vi "TEMP2xxx Control.vi"() -> ()   [LabVIEW 2017]
uses:
  <instrlib>/Samwontech TEMP2xxx/Samwontech TEMP2xxx.lvlib
panel:
  in  "Close port":bool
  in  "Open port":bool
  in  "Exit":bool
  in  "Serial Configuration":T1={"Baud Rate"=9600, "Parity"=0, "Data Bits"=8, "Stop Bits"=10, "Flow Control"=0} {"Flow Control" items=["None", "XON/XOFF", "RTS/CTS", "XON/XOFF & RTS/CTS", "DTR/DSR", "XON/XOFF & DTR/DSR"]; "Stop Bits" items=["1.0"=10, "1.5"=15, "2.0"=20]; "Data Bits" items=["7"=7, "8"=8]; "Parity" items=["None", "Odd", "Even", "Mark", "Space"]; "Baud Rate" items=["300"=300, "600"=600, "1200"=1200, "2400"=2400, "4800"=4800, "9600"=9600, "19200"=19200, "115200"=115200]}
  in  "VISA resource name":refnum<visa-resource-name>
  out "Successfully":bool
  in  "FIX Set Point":dbl format="%1.1f"
  in  "Set Fix Operation Set Point":bool
  out "Successfully":bool
  in  "Run FIX":bool
  in  "Read continuously":bool
  in  "Read Current PV":bool
  out "Data Valid":bool
  out "Current PV":dbl
  out "Responce (original)":string
  out "Successfully":bool
  in  "Data":u32
  in  "Register (write)":u32=1
  in  "Write":bool
  out "Data":u32
  out "Data Valid":bool
  in  "Register (read)":u32=1
  in  "Read":bool
  out "Version-Revision":string
  out "Model Name":string
  in  "AMI":bool
  # "Registers Read/Write:"
  # "FIX Mode Control:"
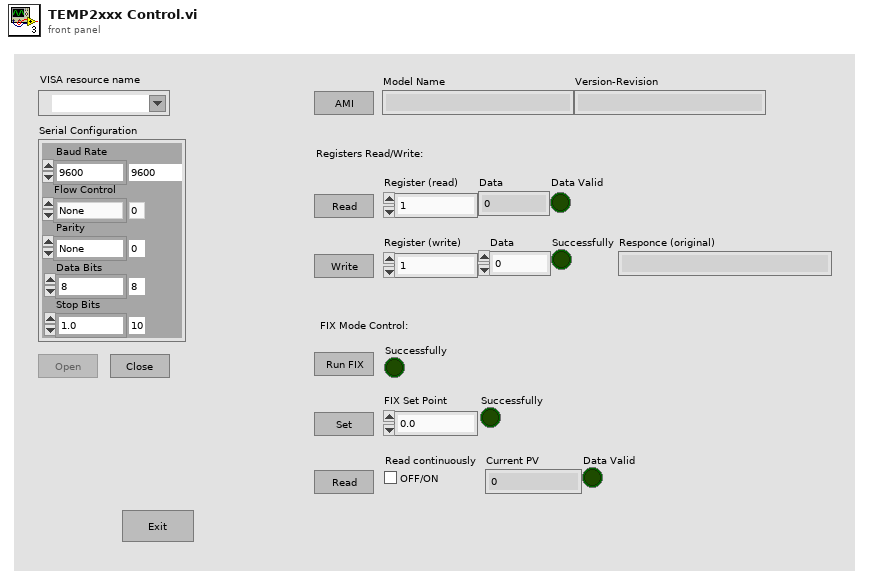
[diagram p1: front panel]
types:
  T1 = cluster{"Baud Rate":u32, "Parity":u16, "Data Bits":u16, "Stop Bits":u16, "Flow Control":u16}
  T2 = enum8{"Enabled", "Disabled", "Disabled and Grayed Out"}
  T3 = enum32{"Invalid", "Standard", "Closed", "Hidden", "Minimized", "Maximized"}
  T4 = enum32{"invalid app kind", "Development System", "Run Time System", "Student Edition", "Embedded LabVIEW", "Evaluation", "Custom"}
  T5 = cluster{"Core":cluster{"Current VI Reference":refnum<vi>, "Close Panel on Exit?":bool}, "Your Boolean data":bool, "Your string data":string, "VISA resource name":refnum<visa-resource-name>, "Is port opened?":bool, "Read: Current PV":bool}
  T6 = cluster{"Current VI Reference":refnum<vi>, "Close Panel on Exit?":bool}
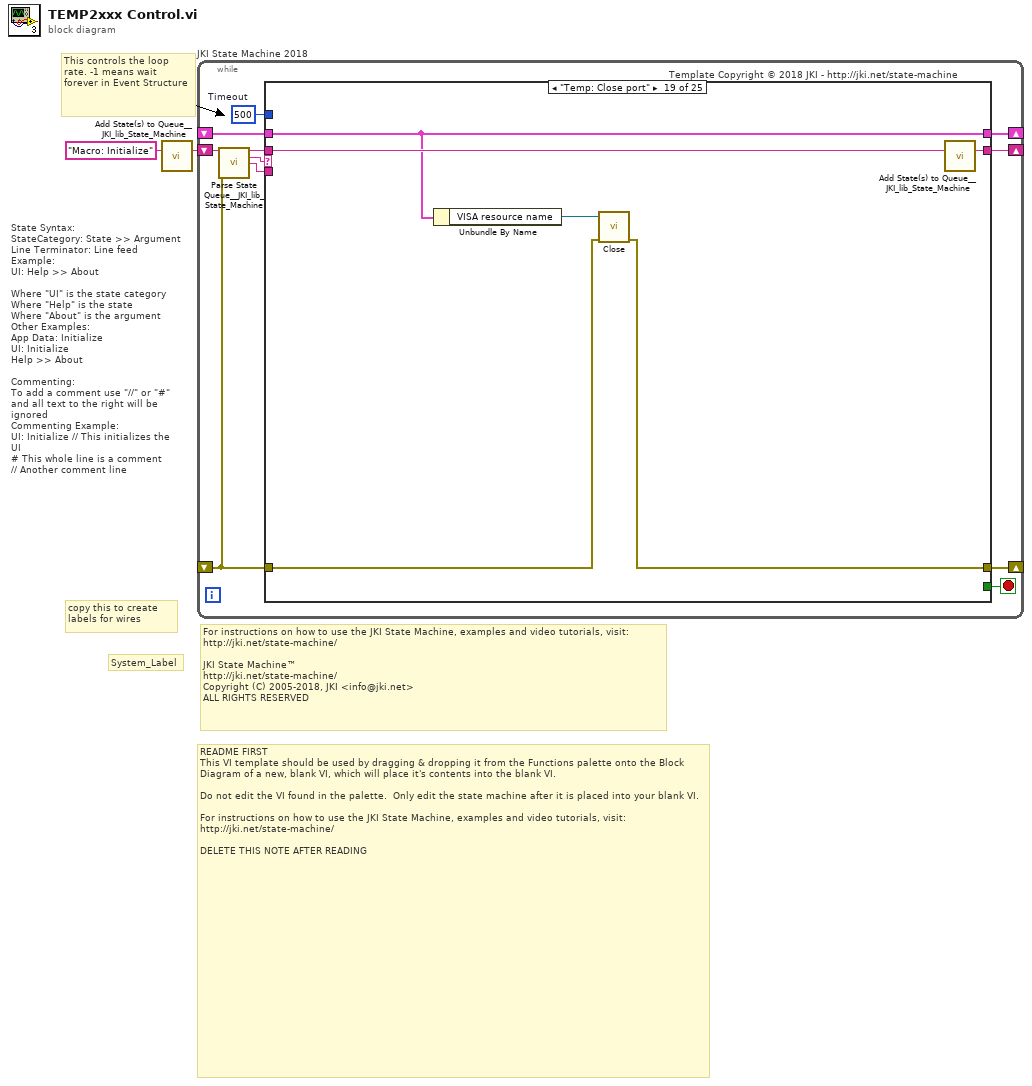
[diagram p0: block diagram]
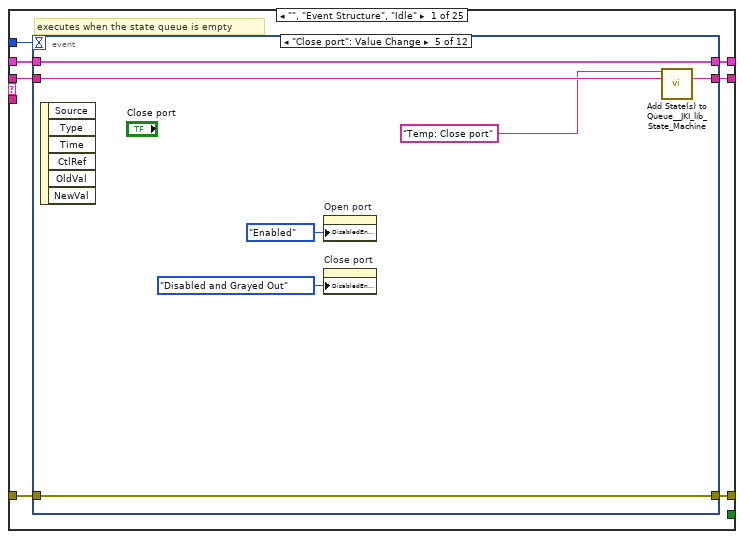
[diagram p2: hidden frame]
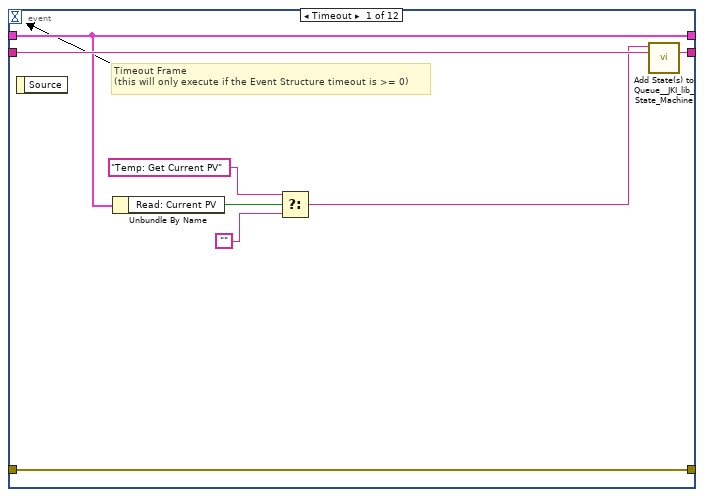
[diagram p3: hidden frame]
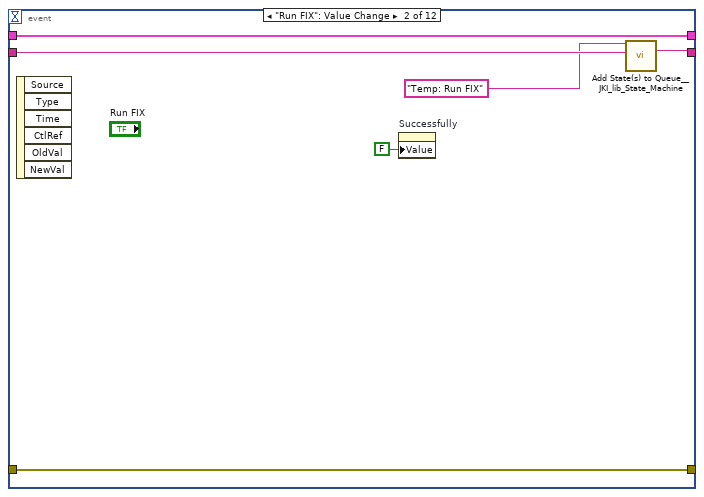
[diagram p4: hidden frame]
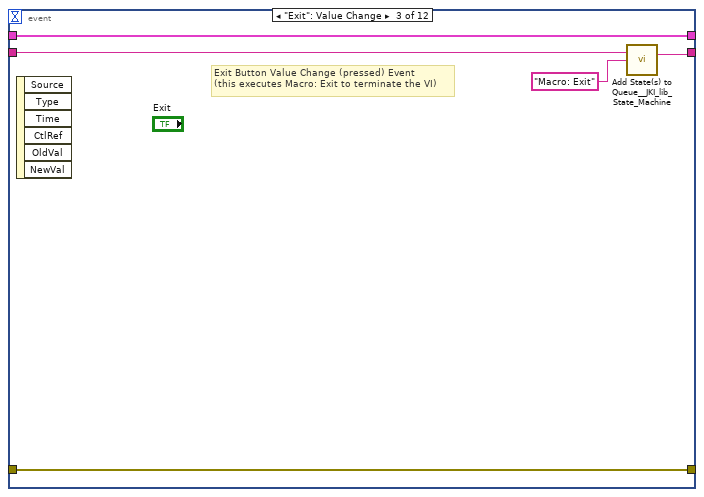
[diagram p5: hidden frame]
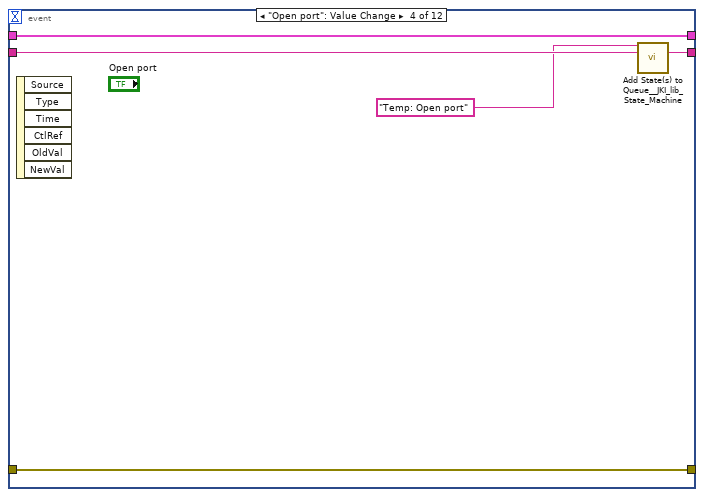
[diagram p6: hidden frame]
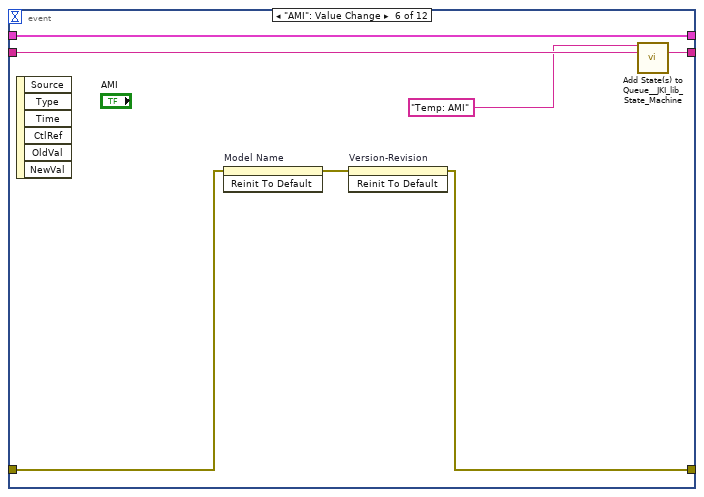
[diagram p7: hidden frame]
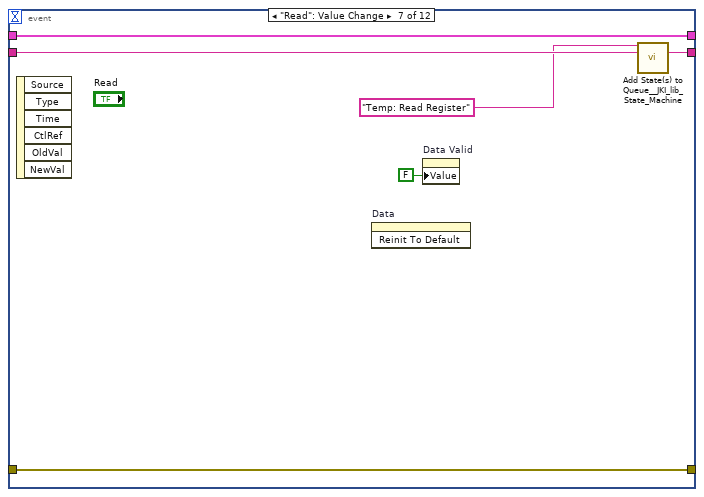
[diagram p8: hidden frame]
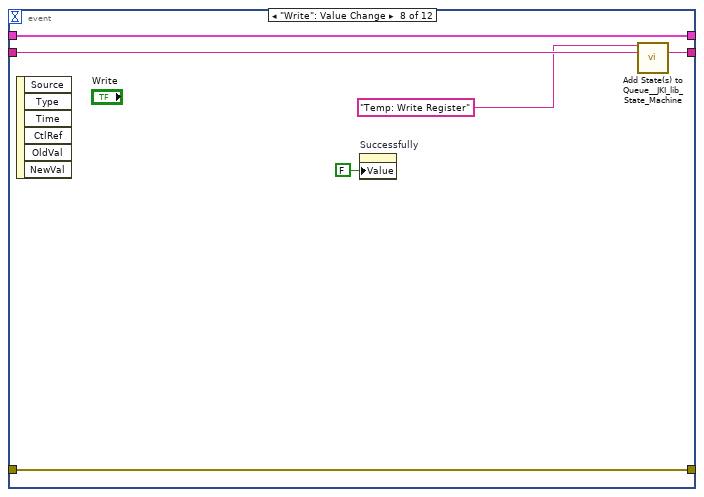
[diagram p9: hidden frame]
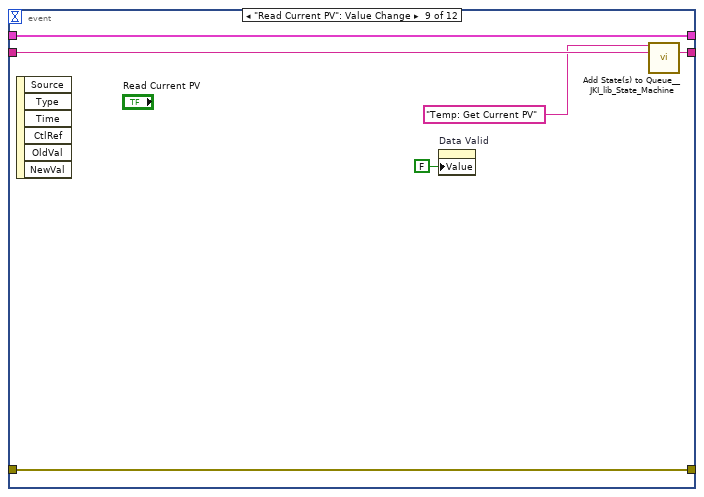
[diagram p10: hidden frame]
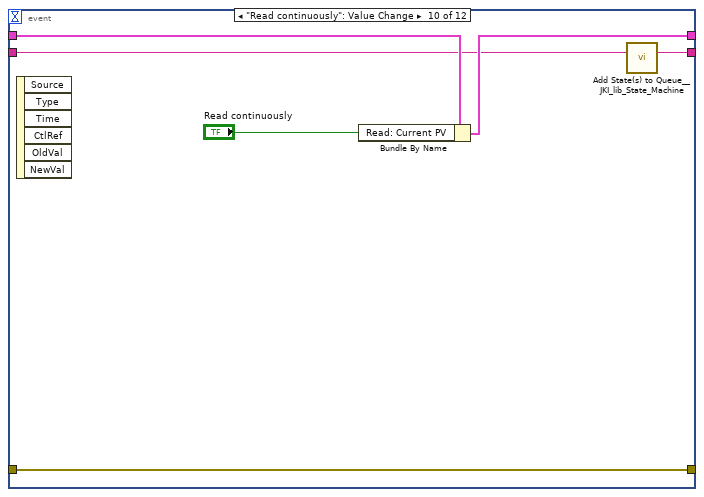
[diagram p11: hidden frame]
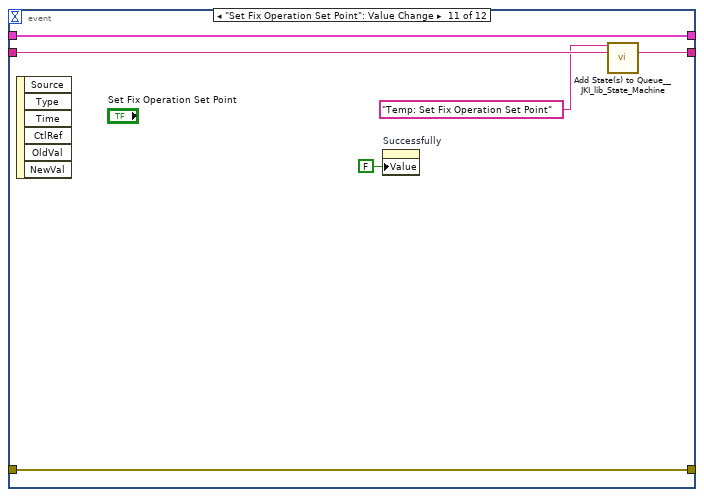
[diagram p12: hidden frame]
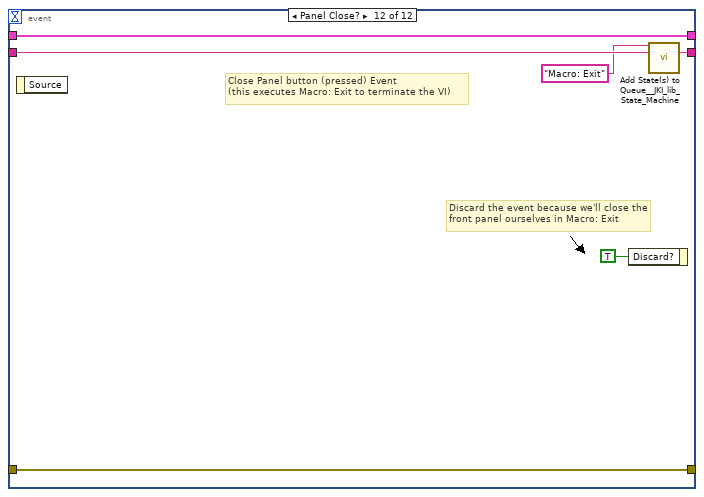
[diagram p13: hidden frame]
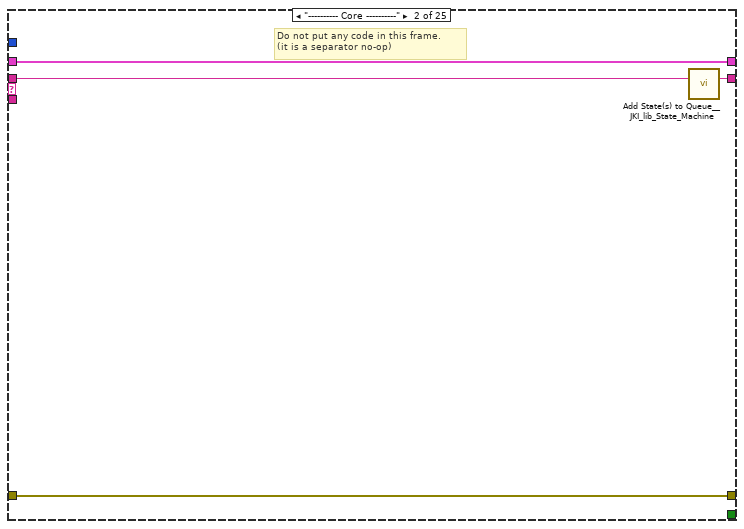
[diagram p14: hidden frame]
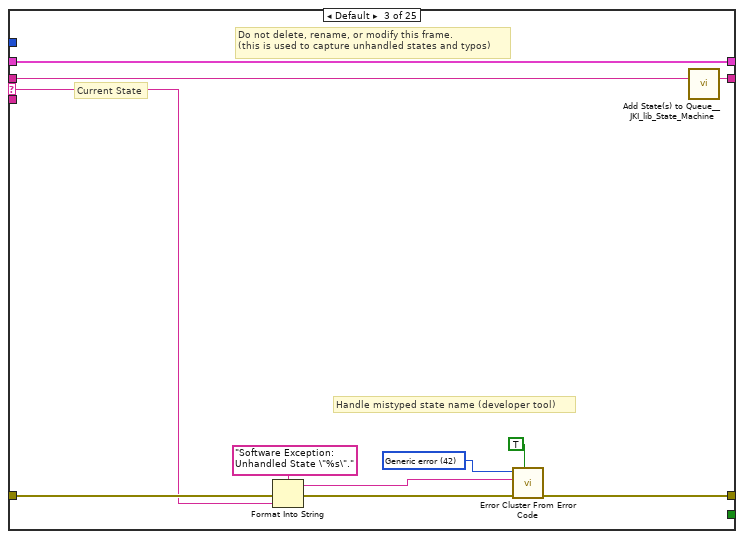
[diagram p15: hidden frame]
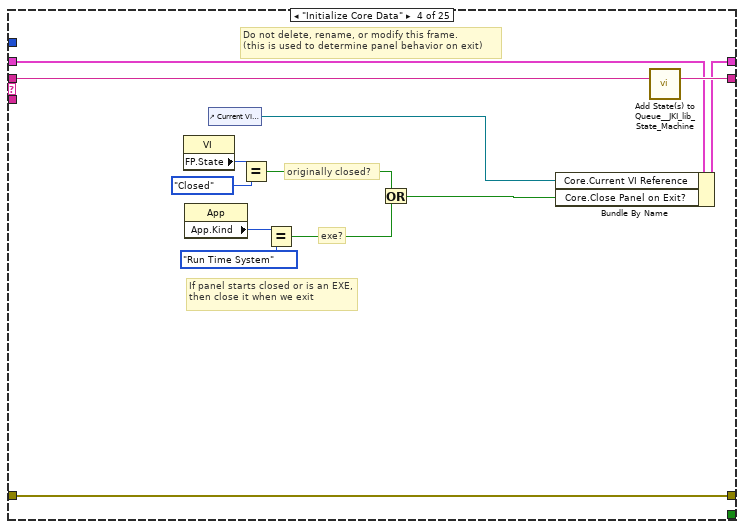
[diagram p16: hidden frame]
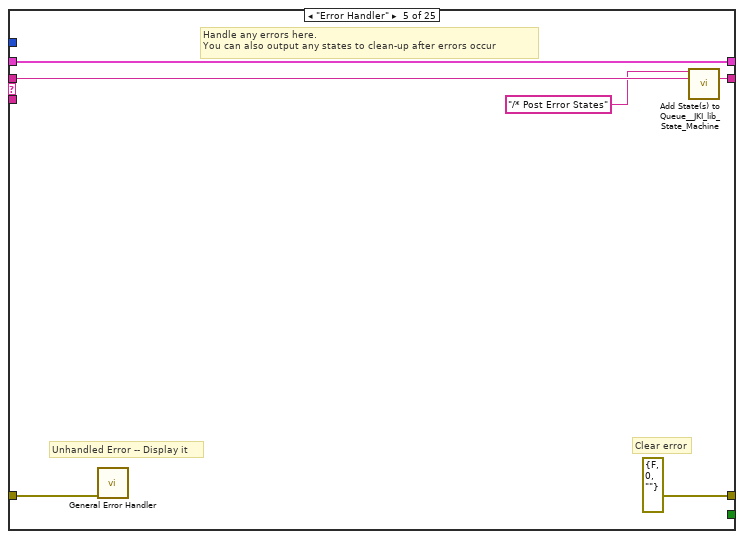
[diagram p17: hidden frame]
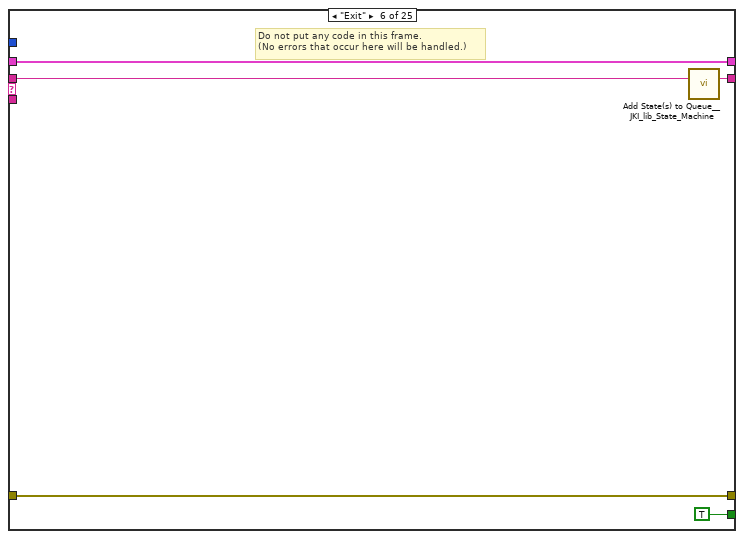
[diagram p18: hidden frame]
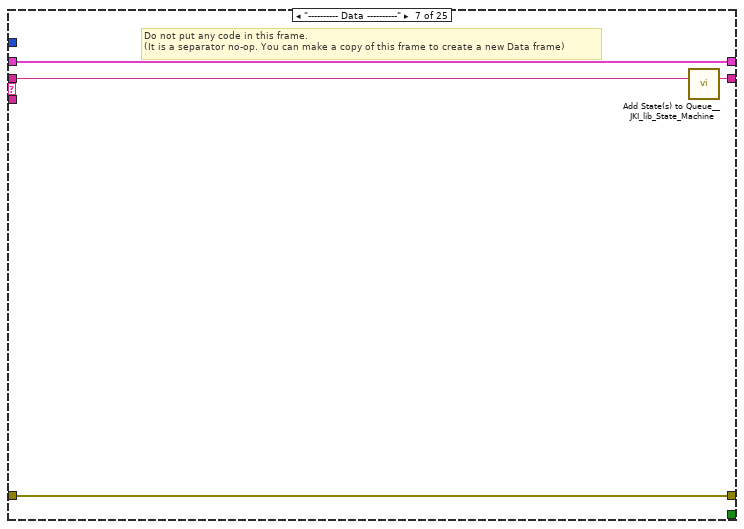
[diagram p19: hidden frame]
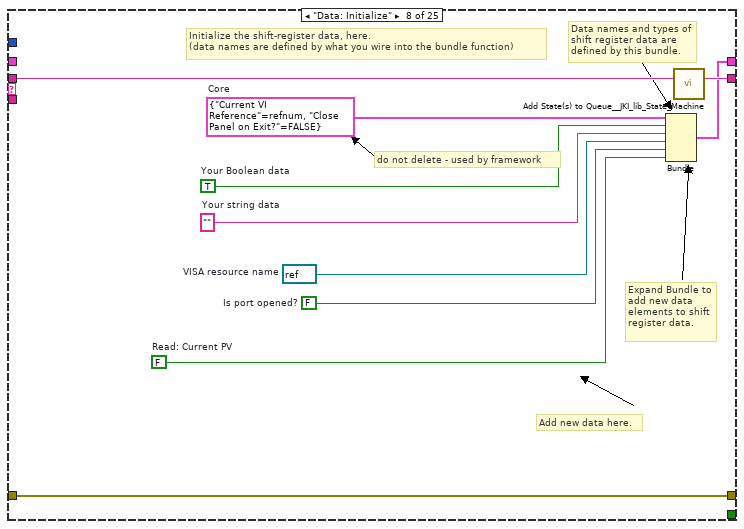
[diagram p20: hidden frame]
diagram:
  # "README FIRST\nThis VI template should be used by dragging & dropping it from the Functions palette onto the Block Diagram of a new, blank VI, which will place it's contents into the blank VI.\n\nDo not edit the VI found in the palette.  Only edit the state machine after it is placed into your blank VI.\n\nFor instructions on how to use the JKI State Machine, examples and video tutorials, visit:\nhttp://jki.net/state-machine/\n\nDELETE THIS NOTE AFTER READING"
  # "For instructions on how to use the JKI State Machine, examples and video tutorials, visit:\nhttp://jki.net/state-machine/\n\nJKI State Machine™\nhttp://jki.net/state-machine/\nCopyright (C) 2005-2018, JKI <info@jki.net>\nALL RIGHTS RESERVED"
  # "State Syntax:\nStateCategory: State >> Argument\nLine Terminator: Line feed\nExample:\nUI: Help >> About\n\nWhere \"UI\" is the state category\nWhere \"Help\" is the state\nWhere \"About\" is the argument\nOther Examples:\nApp Data: Initialize\nUI: Initialize\nHelp >> About\n\nCommenting:\nTo add a comment use \"//\" or \"#\" and all text to the right will be ignored\nCommenting Example:\nUI: Initialize // This initializes the UI\n# This whole line is a comment\n// Another comment line"
  # "copy this to create labels for wires"
  # "This controls the loop rate. -1 means wait forever in Event Structure"
  # "System_Label"
  n1 = call <vilib>:"Add State(s) to Queue__JKI_lib_State_Machine.vi"("State(s) in (\"\")"="Macro: Initialize") -> ("States Out"=w2:string)  [unwired: 14 in]
  n2 = while "JKI State Machine 2018" {
    shift-right: [w6] -> _
    shift-left: _ -> [w5]
    shift-right: [w9] -> _
    shift-left: _ -> [w3]
    shift-right: [w8] -> _
    shift-left: w2 -> [w10]
    stop <- w7 stop-if-true
    w4 = 500  # Timeout
    # "Template Copyright © 2018 JKI - http://jki.net/state-machine"
    n3 = call <vilib>:"Parse State Queue__JKI_lib_State_Machine.vi"("State Queue"=w10, "Error In (no error)"=w3) -> ("Remaining States"=w12:string, "Current State"=w13:string, "Arguments"=w11:string)  [unwired: 11 in]
    n4 = case shown="\"Temp: Close port\"" w13 {
      selector: w13 -> [_ _ w99 _ _ _ _ _ _ _ _ _ _ _ _ _ _ _ _ _ _ _ _ _ _]
      tunnel: w12 -> [w20 w98 w103 w122 w128 w133 w137 w147 w153 w157 w163 w169 w180 w249 w254 w266 w274 w286 w294 w302 w311 w321 w329 w336 w344]
      tunnel: w11 -> [_ _ _ _ _ _ _ _ _ _ _ w164 w174 _ _ _ _ _ _ _ _ _ _ _ _]
      tunnel: w5 -> [w18 w95 w101 w115 w125 w131 w134 _ w148 w154 w161 w167 w176 w246 w251 w263 w271 w281 w292 w300 w309 w319 w327 w334 w342]
      tunnel: [w17 w96 w105 w119 errorcluster {"status"=FALSE, "code"=0, "source"=""} ("error out") w130 w135 w144 w149 w155 w160 w165 w177 w247 w252 w264 w272 w277 w289 w297 w305 w314 w324 w331 w338] -> w9
      tunnel: w3 -> [w16 w96 w104 w119 w124 w130 w135 w144 w150 w155 w160 w166 w178 w247 w252 w264 w272 w279 w290 w298 w306 w315 w325 w332 w339]
      tunnel: [w19 w97 w102 w121 w127 w132 w136 w146 w152 w156 w162 w168 w179 w248 w253 w265 w273 w285 w293 w301 w310 w320 w328 w335 w343] -> w8
      tunnel: [_ _ _ _ _ TRUE _ _ _ _ _ _ _ _ _ _ _ _ _ _ _ _ _ _ _] -> w7
      tunnel: [w15 w95 w101 w120 w125 w131 w134 w145 w148 w154 w161 w167 w176 w246 w251 w263 w271 w280 w292 w300 w309 w319 w327 w334 w342] -> w6
      tunnel: w4 -> [w14 _ _ _ _ _ _ _ _ _ _ _ _ _ _ _ _ _ _ _ _ _ _ _ _]
      frame "", "Event Structure", "Idle" {
        # "executes when the state queue is empty"
        n5 = event shown="[4] \"Close port\": Value Change" {
          selector: _ -> [_ _ _ _ _ _ _ _ _ _ _ _]
          dyn-events: _ -> [_ _ _ _ _ _ _ _ _ _ _ _]
          timeout: w14 -> [_ _ _ _ _ _ _ _ _ _ _ _]
          tunnel: w20 -> [w28 w31 w36 w41 w48 w56 w61 w67 w75 w78 w85 w94]
          tunnel: [w27 w32 w37 w42 w49 w57 w62 w68 w74 w79 w86 w93] -> w19
          tunnel: w18 -> [w25 w33 w38 w43 w50 w58 w63 w69 w76 w81 w87 w91]
          tunnel: [w26 w34 w39 w44 w51 w52 w64 w70 w73 w82 w88 w92] -> w17
          tunnel: w16 -> [w26 w34 w39 w44 w51 w54 w64 w70 w73 w82 w88 w92]
          tunnel: [w25 w33 w38 w43 w50 w58 w63 w69 w76 w80 w87 w91] -> w15
          event Timeout {
            # "Timeout Frame\n(this will only execute if the Event Structure timeout is >= 0)"
            n6 = event-data() -> ()  [unwired: 1 in, 1 out]
            n7 = Unbundle By Name(w25) -> ("Read: Current PV"=w24:bool)
            n8 = Select(t="Temp: Get Current PV", s=w24, f="") -> (s? t:f=w21:string)
            n9 = call <vilib>:"Add State(s) to Queue__JKI_lib_State_Machine.vi"("State(s) in Front (\"\")"=w21, "State(s) in (\"\")"=w28) -> ("States Out"=w27:string)  [unwired: 13 in]
          }
          event "Run FIX": Value Change {
            n10 = event-data() -> ()  [unwired: 1 in, 6 out]
            n11 = property on="Successfully" class="Bool (strict)"("Value"=FALSE ("Successfully")) -> ()  [unwired: 2 in, 2 out]
            n12 = call <vilib>:"Add State(s) to Queue__JKI_lib_State_Machine.vi"("State(s) in Front (\"\")"="Temp: Run FIX", "State(s) in (\"\")"=w31) -> ("States Out"=w32:string)  [unwired: 13 in]
          }
          event "Exit": Value Change {
            # "Exit Button Value Change (pressed) Event\n(this executes Macro: Exit to terminate the VI)"
            n13 = event-data() -> ()  [unwired: 1 in, 6 out]
            n14 = call <vilib>:"Add State(s) to Queue__JKI_lib_State_Machine.vi"("State(s) in (\"\")"=w36, "State(s) at Back (\"\")"="Macro: Exit" ("State(s) at Back (\"\")")) -> ("States Out"=w37:string)  [unwired: 13 in]
          }
          event "Open port": Value Change {
            n15 = event-data() -> ()  [unwired: 1 in, 6 out]
            n16 = call <vilib>:"Add State(s) to Queue__JKI_lib_State_Machine.vi"("State(s) in Front (\"\")"="Temp: Open port" ("State(s) in Front (\"\")"), "State(s) in (\"\")"=w41) -> ("States Out"=w42:string)  [unwired: 13 in]
          }
          event "Close port": Value Change {
            n17 = event-data() -> ()  [unwired: 1 in, 6 out]
            n18 = property on="Open port" class="Bool"("DisabledEnum"=T2."Enabled" ("Disabled")) -> ()  [unwired: 2 in, 2 out]
            n19 = property on="Close port" class="Bool"("DisabledEnum"=T2."Disabled and Grayed Out" ("Disabled")) -> ()  [unwired: 2 in, 2 out]
            n20 = call <vilib>:"Add State(s) to Queue__JKI_lib_State_Machine.vi"("State(s) in Front (\"\")"="Temp: Close port" ("State(s) in Front (\"\")"), "State(s) in (\"\")"=w48) -> ("States Out"=w49:string)  [unwired: 13 in]
          }
          event "AMI": Value Change {
            n21 = event-data() -> ()  [unwired: 1 in, 6 out]
            n22 = invoke on="Model Name" class="Str" method="Reinit To Default"(error in=w54) -> (error out=w53:errorcluster)  [unwired: 2 in, 2 out]
            n23 = invoke on="Version-Revision" class="Str" method="Reinit To Default"(error in=w53) -> (error out=w52:errorcluster)  [unwired: 2 in, 2 out]
            n24 = call <vilib>:"Add State(s) to Queue__JKI_lib_State_Machine.vi"("State(s) in Front (\"\")"="Temp: AMI" ("State(s) in Front (\"\")"), "State(s) in (\"\")"=w56) -> ("States Out"=w57:string)  [unwired: 13 in]
          }
          event "Read": Value Change {
            n25 = event-data() -> ()  [unwired: 1 in, 6 out]
            n26 = invoke on="Data" class="DigNum (strict)" method="Reinit To Default"() -> ()  [unwired: 3 in, 3 out]
            n27 = property on="Data Valid" class="Bool (strict)"("Value"=FALSE ("Data Valid")) -> ()  [unwired: 2 in, 2 out]
            n28 = call <vilib>:"Add State(s) to Queue__JKI_lib_State_Machine.vi"("State(s) in Front (\"\")"="Temp: Read Register" ("State(s) in Front (\"\")"), "State(s) in (\"\")"=w61) -> ("States Out"=w62:string)  [unwired: 13 in]
          }
          event "Write": Value Change {
            n29 = event-data() -> ()  [unwired: 1 in, 6 out]
            n30 = property on="Successfully" class="Bool (strict)"("Value"=FALSE ("Successfully")) -> ()  [unwired: 2 in, 2 out]
            n31 = call <vilib>:"Add State(s) to Queue__JKI_lib_State_Machine.vi"("State(s) in Front (\"\")"="Temp: Write Register" ("State(s) in Front (\"\")"), "State(s) in (\"\")"=w67) -> ("States Out"=w68:string)  [unwired: 13 in]
          }
          event "Read Current PV": Value Change {
            n32 = event-data() -> ()  [unwired: 1 in, 6 out]
            n33 = property on="Data Valid" class="Bool (strict)"("Value"=FALSE ("Data Valid")) -> ()  [unwired: 2 in, 2 out]
            n34 = call <vilib>:"Add State(s) to Queue__JKI_lib_State_Machine.vi"("State(s) in Front (\"\")"="Temp: Get Current PV" ("State(s) in Front (\"\")"), "State(s) in (\"\")"=w75) -> ("States Out"=w74:string)  [unwired: 13 in]
          }
          event "Read continuously": Value Change {
            n35 = event-data() -> ()  [unwired: 1 in, 6 out]
            n36 = Bundle By Name(cluster=w81, "Read: Current PV"="Read continuously") -> (w80:T5)
            n37 = call <vilib>:"Add State(s) to Queue__JKI_lib_State_Machine.vi"("State(s) in (\"\")"=w78) -> ("States Out"=w79:string)  [unwired: 14 in]
          }
          event "Set Fix Operation Set Point": Value Change {
            n38 = event-data() -> ()  [unwired: 1 in, 6 out]
            n39 = property on="Successfully" class="Bool (strict)"("Value"=FALSE ("Successfully")) -> ()  [unwired: 2 in, 2 out]
            n40 = call <vilib>:"Add State(s) to Queue__JKI_lib_State_Machine.vi"("State(s) in Front (\"\")"="Temp: Set Fix Operation Set Point", "State(s) in (\"\")"=w85) -> ("States Out"=w86:string)  [unwired: 13 in]
          }
          event Panel Close? {
            # "Discard the event because we'll close the front panel ourselves in Macro: Exit"
            # "Close Panel button (pressed) Event\n(this executes Macro: Exit to terminate the VI)"
            n41 = event-data() -> ()  [unwired: 1 in, 1 out]
            n42 = event-data("Discard?"=TRUE) -> ()  [unwired: 1 in, 1 out]
            n43 = call <vilib>:"Add State(s) to Queue__JKI_lib_State_Machine.vi"("State(s) in Front (\"\")"="Macro: Exit", "State(s) in (\"\")"=w94) -> ("States Out"=w93:string)  [unwired: 13 in]
          }
        }
      }
      frame "---------- Core ----------" {
        # "Do not put any code in this frame.\n(it is a separator no-op)"
        n44 = call <vilib>:"Add State(s) to Queue__JKI_lib_State_Machine.vi"("State(s) in (\"\")"=w98) -> ("States Out"=w97:string)  [unwired: 14 in]
      }
      frame Default {
        w108 = 42 items=["No error", "Argument error", "Memory is full", "Out of zone", "End of file", "File already open", "Generic file I/O error", "File not found", "File permission error", "Disk is full", "Duplicate path", "Too many files open", "System feature not enabled", "Resource file not found", "Cannot add resource", "Resource not found", "Image not found", "Image memory error", "Pen does not exist", "Config type invalid", "Config token not found", "Config parse error", "Config memory error", "Bad external code format", "Bad external code offset", "External code not present", "Null window", "Destroy window error", "Null menu", "Print aborted", "Bad print record", "Print driver error", "Windows error during printing", "Memory error during printing", "Print dialog error", "Generic print error", "Invalid device refnum", "Device not found", "Device parameter error", "Device unit error", "Cannot open device", "Device call aborted", "Generic error", "Cancelled by user", "Object ID too low", "Object ID too high", "Object not in heap", "Unknown heap", "Unknown object (invalid DefProc)", "Unknown object (DefProc not in table)", "Message out of range", "Invalid (null) method", "Unknown message", "Manager call not supported", "Bad address", "Network operation in progress", "Network operation timed out", "Connection is busy", "Network attribute not supported", "Network error", "Address in use", "System out of memory", "Connection aborted", "Connection refused", "Not connected", "Already connected", "Connection closed", "Initialization error (interapplication manager)", "Bad occurrence", "Wait on unbound occurrence handler", "Occurrence queue overflow", "Datalog type conflict", "Unused", "Unrecognized type (interapplication manager)", "Memory corrupt", "Failed to make temporary DLL", "Old CIN version", "Drag socket not found", "Failed to load drop-object", "Failed to register OLE object", "Failed to release OLE object", "Format specifier type mismatch", "Unknown format specifier", "Too few format specifiers", "Too many format specifiers", "Scan failed", "Newer CIN version", "Error converting to variant", "Runtime menu error", "Password tampered", "Variant attribute not found", "Incompatible variant data type", "Event data is not available", "Event Store is not present", "Occurrence is not found", "Event Queue is not created", "Event info is not available", "Refnum passed is NULL", "Error retrieving Class GUID", "Error retrieving CoClass GUID", "Error retrieving TypeLib GUID.", "Bad built application magic bytes.", "Specific driver is different from the specific driver associated with the Logical Name.", "There is no session opened to the class driver.", "Max Error", "MAX - Error with config objects", "MAX - Error loading configuration", "MAX - Group not supported"]
        # "Current State"
        # "Do not delete, rename, or modify this frame.\n(this is used to capture unhandled states and typos)"
        # "Handle mistyped state name (developer tool)"
        n45 = Format Into String(format string="Software Exception: Unhandled State \"%s\"." ("message"), error in=w104, w99) -> (resulting string=w107:string, error out=w106:errorcluster)  [unwired: 1 in]
        n46 = call <vilib>:"Error Cluster From Error Code.vi"("show call chain? (False)"=TRUE, "error in (no error)"=w106, "error message (\"\")"=w107, "error code (0)"=w108) -> ("error out"=w105:errorcluster)  [unwired: 5 in]
        n47 = call <vilib>:"Add State(s) to Queue__JKI_lib_State_Machine.vi"("State(s) in (\"\")"=w103) -> ("States Out"=w102:string)  [unwired: 14 in]
      }
      frame "Initialize Core Data" {
        # "Do not delete, rename, or modify this frame.\n(this is used to determine panel behavior on exit)"
        # "originally closed?"
        # "exe?"
        # "If panel starts closed or is an EXE, then close it when we exit"
        n48 = property class="VI"() -> ("FP.State"=w112:T3)  [unwired: 2 in, 2 out]
        n49 = property class="App"() -> ("App.Kind"=w118:T4)  [unwired: 2 in, 2 out]
        n50 = control-ref of="Current VI Reference"() -> (w113:refnum<vi>)
        n51 = Equal?(x=w112, y=T3."Closed" ("Front Panel Window:State")) -> (x = y?=w110:bool)
        n52 = Equal?(x=w118, y=T4."Run Time System" ("Application:Kind")) -> (x = y?=w116:bool)
        n53 = Or(x=w110, y=w116) -> (x .or. y?=w114:bool)
        n54 = Bundle By Name(cluster=w115, "Core.Current VI Reference"=w113, "Core.Close Panel on Exit?"=w114) -> (w120:T5)
        n55 = call <vilib>:"Add State(s) to Queue__JKI_lib_State_Machine.vi"("State(s) in (\"\")"=w122) -> ("States Out"=w121:string)  [unwired: 14 in]
      }
      frame "Error Handler" {
        # "Unhandled Error -- Display it"
        # "Handle any errors here.\nYou can also output any states to clean-up after errors occur"
        # "Clear error"
        n56 = call <vilib>:"General Error Handler.vi"("error in (no error)"=w124) -> ()  [unwired: 10 in, 5 out]
        n57 = call <vilib>:"Add State(s) to Queue__JKI_lib_State_Machine.vi"("State(s) in Front (\"\")"="/* Post Error States", "State(s) in (\"\")"=w128) -> ("States Out"=w127:string)  [unwired: 13 in]
      }
      frame "Exit" {
        # "Do not put any code in this frame.\n(No errors that occur here will be handled.)"
        n58 = call <vilib>:"Add State(s) to Queue__JKI_lib_State_Machine.vi"("State(s) in (\"\")"=w133) -> ("States Out"=w132:string)  [unwired: 14 in]
      }
      frame "---------- Data ----------" {
        # "Do not put any code in this frame.\n(It is a separator no-op. You can make a copy of this frame to create a new Data frame)"
        n59 = call <vilib>:"Add State(s) to Queue__JKI_lib_State_Machine.vi"("State(s) in (\"\")"=w137) -> ("States Out"=w136:string)  [unwired: 14 in]
      }
      frame "Data: Initialize" {
        w138 = FALSE  # Read: Current PV
        w139 = FALSE  # Is port opened?
        w140 = refnum<visa-resource-name> refnum  # VISA resource name
        w141 = T6 {"Current VI Reference"=refnum, "Close Panel on Exit?"=FALSE}  # Core
        w143 = TRUE  # Your Boolean data
        w142 = ""  # Your string data
        # "do not delete - used by framework"
        # "Expand Bundle to add new data elements to shift register data."
        # "Add new data here."
        # "Data names and types of shift register data are defined by this bundle."
        # "Initialize the shift-register data, here.\n(data names are defined by what you wire into the bundle function)"
        n60 = Bundle("Core"=w141, "Your Boolean data"=w143, "Your string data"=w142, "VISA resource name"=w140, "Is port opened?"=w139, "Read: Current PV"=w138) -> (w145:T5)  [unwired: 1 in]
        n61 = call <vilib>:"Add State(s) to Queue__JKI_lib_State_Machine.vi"("State(s) in (\"\")"=w147) -> ("States Out"=w146:string)  [unwired: 14 in]
      }
      frame "Data: Cleanup" {
        # "Cleanup any data and references, here.\n(this is called automatically, by the Macro: Exit)"
        n62 = Unbundle By Name(w148) -> ("Core.Current VI Reference"=w151:refnum<vi>)
        n63 = Close Reference(reference=w151, error in (no error)=w150) -> (error out=w149:errorcluster)
        n64 = call <vilib>:"Add State(s) to Queue__JKI_lib_State_Machine.vi"("State(s) in (\"\")"=w153) -> ("States Out"=w152:string)  [unwired: 14 in]
      }
      frame "---------- UI ----------" {
        # "Do not put any code in this frame.\n(It is a separator no-op. You can make a copy of this frame to create a new UI frame)"
        n65 = call <vilib>:"Add State(s) to Queue__JKI_lib_State_Machine.vi"("State(s) in (\"\")"=w157) -> ("States Out"=w156:string)  [unwired: 14 in]
      }
      frame "UI: Initialize" {
        # "Initialize the User Interface, here.\n(this is called automatically, by the Macro: Init)"
        n66 = property on="Open port" class="Bool"("DisabledEnum"=T2."Enabled" ("Disabled")) -> ()  [unwired: 2 in, 2 out]
        n67 = property on="Close port" class="Bool"("DisabledEnum"=T2."Disabled and Grayed Out" ("Disabled")) -> ()  [unwired: 2 in, 2 out]
        n68 = call <vilib>:"Add State(s) to Queue__JKI_lib_State_Machine.vi"("State(s) in (\"\")"=w163) -> ("States Out"=w162:string)  [unwired: 14 in]
      }
      frame "UI: Cursor Set" {
        # "Argument"
        # "Set and Unset Cursor Busy.\n(Usage: \"UI: Cursor Set >> Busy|Idle\")"
        n69 = case shown="\"Idle\", Default" w164 {
          tunnel: w166 -> [w171 w173]
          tunnel: [w170 w172] -> w165
          frame "Idle", Default {
            n70 = call <vilib>:"Unset Busy.vi"("error in (no error)"=w171) -> ("error out"=w170:errorcluster)  [unwired: 10 in]
          }
          frame "Busy" {
            n71 = call <vilib>:"Set Busy.vi"("error in (no error)"=w173) -> ("error out"=w172:errorcluster)  [unwired: 9 in, 1 out]
          }
        }
        n72 = call <vilib>:"Add State(s) to Queue__JKI_lib_State_Machine.vi"("State(s) in (\"\")"=w169) -> ("States Out"=w168:string)  [unwired: 14 in]
      }
      frame "UI: Front Panel State" {
        # "Argument"
        # "Set Front Panel Open or Closed\n(Usage: \"UI: Front Panel State >> Open|Close\")"
        n73 = Unbundle By Name(w176) -> ("Core.Current VI Reference"=w175:refnum<vi>)
        n74 = case shown="\"Minimize\", \"Minimized\"" w174 {
          tunnel: w178 -> [w186 w201 w212 w225 w238]
          tunnel: [w188 w202 w214 w227 w240] -> w177
          tunnel: w175 -> [w187 w199 w213 w226 w239]
          frame "Open", "Standard", Default {
            w181 = T3."Standard" ("State")
            n75 = property class="VI"(reference=w187, error in=w186) -> (reference out=w184:refnum<vi>, error out=w185:errorcluster, "FP.State"=w183:T3)
            n76 = Not Equal?(x=w183, y=w181) -> (x != y?=w182:bool)
            n77 = case shown="True" w182 {
              tunnel: [w192 w194] -> w188
              tunnel: w185 -> [w191 w194]
              tunnel: w184 -> [w190 _]
              tunnel: w181 -> [w189 _]
              frame True {
                n78 = invoke class="VI" method="FP.Open"(reference=w190, error in=w191, "Activate"=TRUE, "State"=w189) -> (error out=w192:errorcluster)  [unwired: 1 in, 4 out]
              }
              frame False {
              }
            }
          }
          frame "Close", "Closed" {
            n79 = property class="VI"(reference=w199, error in=w201) -> (reference out=w198:refnum<vi>, error out=w200:errorcluster, "FP.State"=w196:T3)
            n80 = Not Equal?(x=w196, y=T3."Closed" ("Front Panel Window:State")) -> (x != y?=w195:bool)
            n81 = case shown="True" w195 {
              tunnel: [w203 w206] -> w202
              tunnel: w200 -> [w203 w205]
              tunnel: w198 -> [_ w204]
              frame False {
              }
              frame True {
                n82 = invoke class="VI" method="FP.Close"(reference=w204, error in=w205) -> (error out=w206:errorcluster)  [unwired: 1 in, 2 out]
              }
            }
          }
          frame "Hidden", "Hide" {
            w207 = T3."Hidden" ("State")
            n83 = property class="VI"(reference=w213, error in=w212) -> (reference out=w210:refnum<vi>, error out=w211:errorcluster, "FP.State"=w209:T3)
            n84 = Not Equal?(x=w209, y=w207) -> (x != y?=w208:bool)
            n85 = case shown="True" w208 {
              tunnel: [w218 w219] -> w214
              tunnel: w211 -> [w217 w219]
              tunnel: w210 -> [w216 _]
              tunnel: w207 -> [w215 _]
              frame True {
                n86 = invoke class="VI" method="FP.Open"(reference=w216, error in=w217, "State"=w215) -> (error out=w218:errorcluster)  [unwired: 2 in, 4 out]
              }
              frame False {
              }
            }
          }
          frame "Minimize", "Minimized" {
            w220 = T3."Minimized" ("State")
            n87 = property class="VI"(reference=w226, error in=w225) -> (reference out=w223:refnum<vi>, error out=w224:errorcluster, "FP.State"=w222:T3)
            n88 = Not Equal?(x=w222, y=w220) -> (x != y?=w221:bool)
            n89 = case shown="True" w221 {
              tunnel: [w231 w232] -> w227
              tunnel: w224 -> [w230 w232]
              tunnel: w223 -> [w229 _]
              tunnel: w220 -> [w228 _]
              frame True {
                n90 = invoke class="VI" method="FP.Open"(reference=w229, error in=w230, "State"=w228) -> (error out=w231:errorcluster)  [unwired: 2 in, 4 out]
              }
              frame False {
              }
            }
          }
          frame "Maximize", "Maximized" {
            w233 = T3."Maximized" ("State")
            n91 = property class="VI"(reference=w239, error in=w238) -> (reference out=w236:refnum<vi>, error out=w237:errorcluster, "FP.State"=w235:T3)
            n92 = Not Equal?(x=w235, y=w233) -> (x != y?=w234:bool)
            n93 = case shown="True" w234 {
              tunnel: [w244 w245] -> w240
              tunnel: w237 -> [w243 w245]
              tunnel: w236 -> [w242 _]
              tunnel: w233 -> [w241 _]
              frame True {
                n94 = invoke class="VI" method="FP.Open"(reference=w242, error in=w243, "State"=w241) -> (error out=w244:errorcluster)  [unwired: 2 in, 4 out]
              }
              frame False {
              }
            }
          }
        }
        n95 = call <vilib>:"Add State(s) to Queue__JKI_lib_State_Machine.vi"("State(s) in (\"\")"=w180) -> ("States Out"=w179:string)  [unwired: 14 in]
      }
      frame "---------- Macro ----------" {
        # "Do not put any code in this frame.\n(It is a separator no-op. You can make a copy of this frame to create a new Macro frame)"
        n96 = call <vilib>:"Add State(s) to Queue__JKI_lib_State_Machine.vi"("State(s) in (\"\")"=w249) -> ("States Out"=w248:string)  [unwired: 14 in]
      }
      frame "Macro: Initialize" {
        w250 = "Data: Initialize\nInitialize Core Data\nUI: Initialize\nUI: Front Panel State >> Open"  # Data: Initialize Initialize Core Data UI: Initialize UI: Front Panel State >> Open
        # "Initialization Macro\n(This is called once, when the VI starts)"
        n97 = call <vilib>:"Add State(s) to Queue__JKI_lib_State_Machine.vi"("State(s) in Front (\"\")"=w250, "State(s) in (\"\")"=w254) -> ("States Out"=w253:string)  [unwired: 13 in]
      }
      frame "Macro: Exit" {
        # "Exit Macro\n(This is called once, when the VI exits)"
        n98 = Unbundle By Name(w263) -> ("Core.Close Panel on Exit?"=w262:bool, "Is port opened?"=w256:bool)
        n99 = Select(t="UI: Front Panel State >> Close", s=w262, f="") -> (s? t:f=w257:string)
        n100 = case shown="True" w256 {
          tunnel: w257 -> [w267 w270]
          tunnel: [w267 w269] -> w255
          frame False {
          }
          frame True {
            n101 = call <vilib>:"Add State(s) to Queue__JKI_lib_State_Machine.vi"("State(s) in Front (\"\")"=w270, "State(s) in (\"\")"="Temp: Close port") -> ("States Out"=w269:string)  [unwired: 13 in]
          }
        }
        n102 = call <vilib>:"Add State(s) to Queue__JKI_lib_State_Machine.vi"("State(s) in (\"\")"=w255, "State(s) at Back (\"\")"="Data: Cleanup\nExit") -> ("States Out"=w258:string)  [unwired: 13 in]
        n103 = call <vilib>:"Add State(s) to Queue__JKI_lib_State_Machine.vi"("State(s) in Front (\"\")"=w258, "State(s) in (\"\")"=w266) -> ("States Out"=w265:string)  [unwired: 13 in]
      }
      frame "---------- TEMP Control ----------" {
        # "Template Separator\n(You can make a copy of, or modify, this frame)"
        n104 = call <vilib>:"Add State(s) to Queue__JKI_lib_State_Machine.vi"("State(s) in (\"\")"=w274) -> ("States Out"=w273:string)  [unwired: 14 in]
      }
      frame "Temp: Open port" {
        n105 = call <instrlib>:"Initialize.vi"("Serial Configuration"="Serial Configuration", "error in (no error)"=w279, "ID Query (True)"=FALSE, "VISA resource name"="VISA resource name") -> ("error out"=w277:errorcluster, "VISA resource name out"=w278:refnum<visa-resource-name>)  [unwired: 6 in]
        n106 = Unbundle By Name(w277) -> ("status"=w276:bool)
        n107 = Not(x=w276) -> (.not. x?=w275:bool)
        n108 = case shown="True" w275 {
          frame False {
          }
          frame True {
            n109 = property on="Open port" class="Bool"("DisabledEnum"=T2."Disabled and Grayed Out" ("Disabled")) -> ()  [unwired: 2 in, 2 out]
            n110 = property on="Close port" class="Bool"("DisabledEnum"=T2."Enabled" ("Disabled")) -> ()  [unwired: 2 in, 2 out]
          }
        }
        n111 = Bundle By Name(cluster=w281, "VISA resource name"=w278, "Is port opened?"=w275) -> (w280:T5)
        n112 = call <vilib>:"Add State(s) to Queue__JKI_lib_State_Machine.vi"("State(s) in (\"\")"=w286) -> ("States Out"=w285:string)  [unwired: 14 in]
      }
      frame "Temp: Close port" {
        n113 = Unbundle By Name(w292) -> ("VISA resource name"=w291:refnum<visa-resource-name>)
        n114 = call <instrlib>:"Close.vi"("error in (no error)"=w290, "VISA resource name"=w291) -> ("error out"=w289:errorcluster)  [unwired: 9 in]
        n115 = call <vilib>:"Add State(s) to Queue__JKI_lib_State_Machine.vi"("State(s) in (\"\")"=w294) -> ("States Out"=w293:string)  [unwired: 14 in]
      }
      frame "Temp: AMI" {
        n116 = Unbundle By Name(w300) -> ("VISA resource name"=w299:refnum<visa-resource-name>)
        n117 = call <instrlib>:"AMI.vi"("VISA resource name"=w299, "error in"=w298) -> ("Model Name"=→"Model Name":string, "Version-Revision"=→"Version-Revision":string, "error out"=w297:errorcluster)  [unwired: 8 in, 3 out]
        n118 = call <vilib>:"Add State(s) to Queue__JKI_lib_State_Machine.vi"("State(s) in (\"\")"=w302) -> ("States Out"=w301:string)  [unwired: 14 in]
      }
      frame "Temp: Read Register" {
        n119 = Unbundle By Name(w309) -> ("VISA resource name"=w308:refnum<visa-resource-name>)
        n120 = call <instrlib>:"Read D-Register.vi"("error in"=w306, "D-register number"="Register (read)", "VISA resource name"=w308) -> ("error out"=w305:errorcluster, "Data"=→"Data":u32, "Data Valid"=→"Data Valid":bool)  [unwired: 4 in, 2 out]
        n121 = call <vilib>:"Add State(s) to Queue__JKI_lib_State_Machine.vi"("State(s) in (\"\")"=w311) -> ("States Out"=w310:string)  [unwired: 14 in]
      }
      frame "Temp: Write Register" {
        n122 = Unbundle By Name(w319) -> ("VISA resource name"=w318:refnum<visa-resource-name>)
        n123 = call <instrlib>:"Write D-Register.vi"("error in"=w315, "Data"="Data", "D-register number"="Register (write)", "VISA resource name"=w318) -> ("error out"=w314:errorcluster, "Successfully"=→"Successfully":bool, "Responce (original)"=→"Responce (original)":string)  [unwired: 4 in, 1 out]
        n124 = call <vilib>:"Add State(s) to Queue__JKI_lib_State_Machine.vi"("State(s) in (\"\")"=w321) -> ("States Out"=w320:string)  [unwired: 14 in]
      }
      frame "Temp: Get Current PV" {
        n125 = Unbundle By Name(w327) -> ("VISA resource name"=w326:refnum<visa-resource-name>)
        n126 = call <instrlib>:"Get Current PV.vi"("error in"=w325, "VISA resource name"=w326) -> ("error out"=w324:errorcluster, "Current PV"=→"Current PV":dbl, "Data Valid"=→"Data Valid":bool)  [unwired: 6 in, 1 out]
        n127 = call <vilib>:"Add State(s) to Queue__JKI_lib_State_Machine.vi"("State(s) in (\"\")"=w329) -> ("States Out"=w328:string)  [unwired: 14 in]
      }
      frame "Temp: Run FIX" {
        n128 = Unbundle By Name(w334) -> ("VISA resource name"=w333:refnum<visa-resource-name>)
        n129 = call <instrlib>:"Run Fix Operation.vi"("error in"=w332, "VISA resource name"=w333) -> ("error out"=w331:errorcluster, "Successfully"=→"Successfully":bool)  [unwired: 7 in, 1 out]
        n130 = call <vilib>:"Add State(s) to Queue__JKI_lib_State_Machine.vi"("State(s) in (\"\")"=w336) -> ("States Out"=w335:string)  [unwired: 14 in]
      }
      frame "Temp: Set Fix Operation Set Point" {
        n131 = Unbundle By Name(w342) -> ("VISA resource name"=w341:refnum<visa-resource-name>)
        n132 = call <instrlib>:"Set Fix Operation Set Point.vi"("error in"=w339, "Set Point"="FIX Set Point", "VISA resource name"=w341) -> ("error out"=w338:errorcluster, "Successfully"=→"Successfully":bool)  [unwired: 6 in, 1 out]
        n133 = call <vilib>:"Add State(s) to Queue__JKI_lib_State_Machine.vi"("State(s) in (\"\")"=w344) -> ("States Out"=w343:string)  [unwired: 14 in]
      }
    }
  }
